vi "FTW-Connector-Ask.vi"(0 "FTW Actor Connector":refnum<class "FTW-ActorConnector.lvclass">, 5 "Request Header":string, 7 "Request Body":string, 9 "Timeout":i32=1000 format="%dmsec", 11 "error in":errorcluster) -> (4 "FTW Actor Connector out":refnum<class "FTW-ActorConnector.lvclass">, 6 "Response Header":string, 8 "Response Body":string, 10 "Timed out?":bool, 13 "Response Metadata":string, 14 "Roundtrip Time":dbl format="%.6fsec", 15 "error out":errorcluster)   [LabVIEW 2013, in "FTW-ActorConnector.lvclass"]
uses:
  FTW-ActorConnector.lvclass
  FTW-ActorConnector.lvclass/FTW-ActorConnector.ctl
  Request/FTW-Request.lvclass
panel:
  # "Inputs"
  # "Outputs"
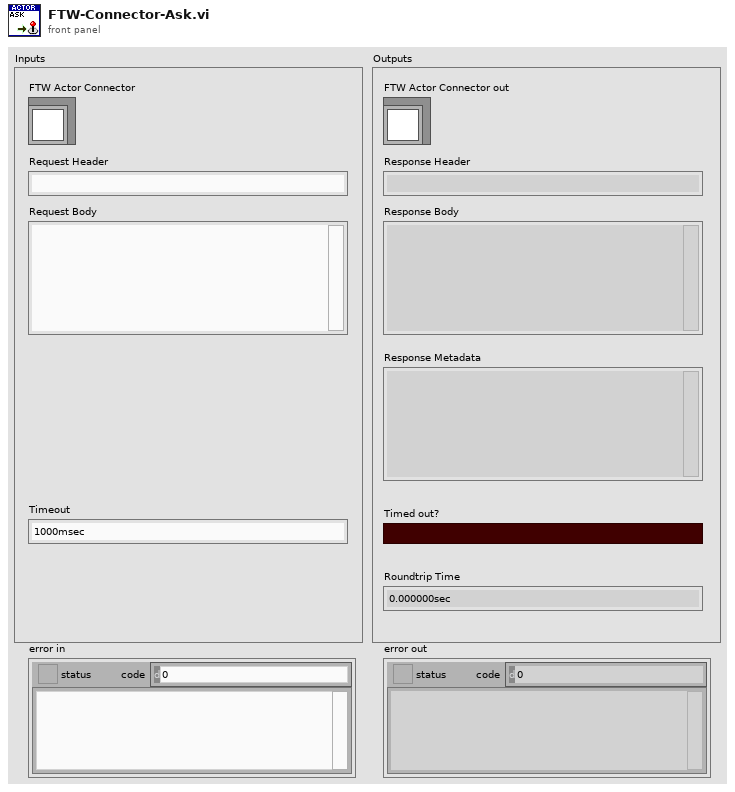
[diagram p1: front panel]
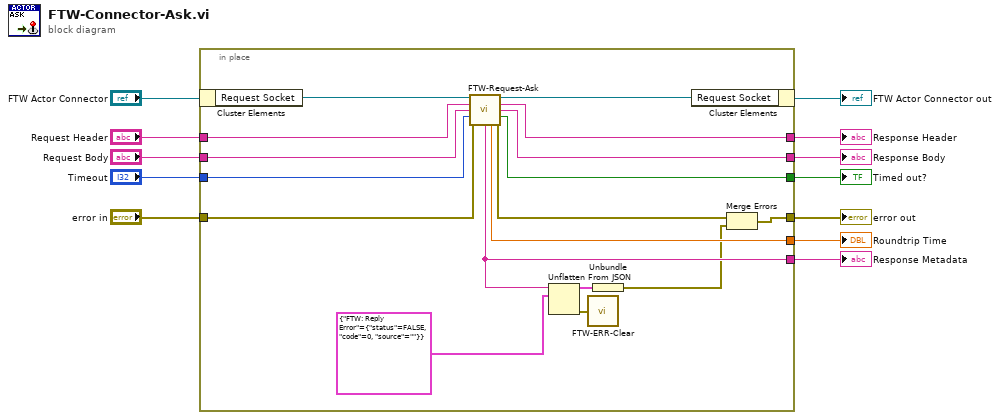
[diagram p0: block diagram]
diagram:
  n1 = in-place {
    in-place-border: "error in" -> [w29]
    in-place-border: [w14] -> w11
    in-place-border: "Request Header" -> [w24]
    in-place-border: "Request Body" -> [w23]
    in-place-border: [w25] -> w8
    in-place-border: "Timeout" -> [w22]
    in-place-border: [w21] -> w4
    in-place-border: [w20] -> w3
    in-place-border: [w19] -> w2
    in-place-border: [w16] -> w1
    n2 = in-place-cluster #1("FTW Actor Connector") -> ("Request Socket"=w27:refnum<class "FTW-Request.lvclass">)
    n3 = call "FTW-Request-Ask.vi"("FTW-Request In"=w27, "Header"=w24, "Body"=w23, "Timeout"=w22, "error in"=w29) -> ("FTW-Request Out"=w26:refnum<class "FTW-Request.lvclass">, "Response Header"=w21:string, "Response Body"=w20:string, "Timed out?"=w25:bool, "Response Metadata"=w16:string, "Roundtrip Time"=w19:dbl, "error out"=w28:errorcluster)  [unwired: 4 in]
    n4 = Unflatten From JSON(JSON string=w16, type and defaults=cluster{"FTW: Reply Error":errorcluster} {"FTW: Reply Error"={"status"=FALSE, "code"=0, "source"=""}} ("cluster")) -> (value=w15:cluster{"FTW: Reply Error":errorcluster}, error out=w17:errorcluster)  [unwired: 5 in]
    n5 = call "FTW-ERR-Clear.vi"("error to snuff"=w17) -> ()  [unwired: 1 out]
    n6 = Unbundle(w15) -> ("FTW: Reply Error"=w13:errorcluster)
    n7 = in-place-cluster #1("Request Socket"=w26) -> (→"FTW Actor Connector out":refnum<class "FTW-ActorConnector.lvclass">)
    n8 = Merge Errors(w28, w13) -> (w14:errorcluster)
  }
  "error out" <- w11
  "Timed out?" <- w8
  "Response Header" <- w4
  "Response Body" <- w3
  "Roundtrip Time" <- w2
  "Response Metadata" <- w1
